vi "4_2_match_per_line.vi"(11 "String":string) -> (1 "Numeric":i32, 3 "match substring":string)   [LabVIEW 2021, in "2023.lvlib"]
uses:
  2023.lvlib
  Program Files (x86)/National Instruments/LabVIEW 2023/user.lib/_OpenG.lib/array/array.llb/Search 1D Array (I32)__ogtk.vi
  Program Files (x86)/National Instruments/LabVIEW 2023/user.lib/_OpenG.lib/array/array.llb/Delete Elements from 1D Array (I32)__ogtk.vi
  Program Files (x86)/National Instruments/LabVIEW 2023/user.lib/_OpenG.lib/array/array.llb/Remove Duplicates from 1D Array (I32)__ogtk.vi
panel:
  out "array w/ subset deleted":i32[](array[numeric])
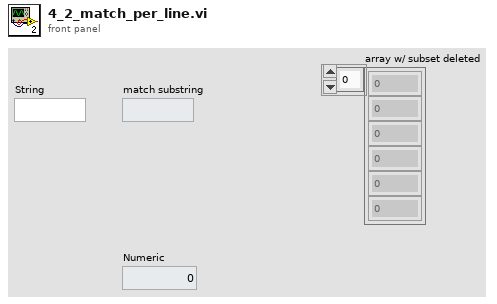
[diagram p1: front panel]
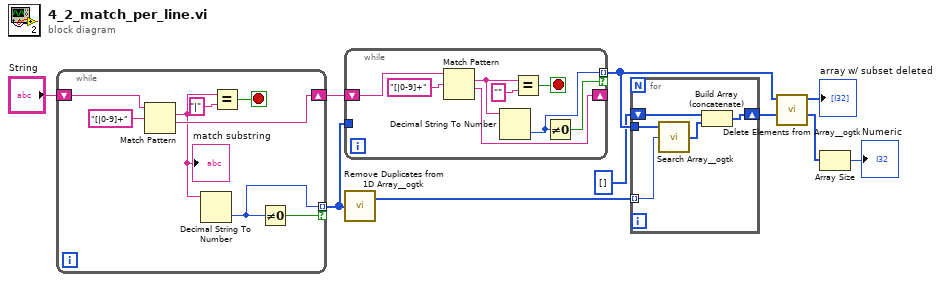
[diagram p0: block diagram]
diagram:
  n1 = while {
    shift-right: [w16] -> w3
    shift-left: "String" -> [w17]
    tunnel: [w12] -> w8 mode=indexing if=w11
    stop <- w13 stop-if-true
    n2 = Match Pattern(string=w17, regular expression="[|0-9]+") -> (match substring=w14:string, after substring=w16:string)  [unwired: 1 in, 2 out]
    "match substring" <- w14
    n3 = Decimal String To Number(string=w14) -> (number=w12:i32)  [unwired: 2 in, 1 out]
    n4 = Equal?(x=w14, y="|") -> (x = y?=w13:bool)
    n5 = Not Equal To 0?(x=w12) -> (x != 0?=w11:bool)
  }
  n6 = while {
    shift-right: [w24] -> _
    shift-left: w3 -> [w25]
    tunnel: [w19] -> w7 mode=indexing if=w20
    tunnel: w8 -> [_]
    stop <- w21 stop-if-true
    n7 = Match Pattern(string=w25, regular expression="[|0-9]+") -> (match substring=w22:string, after substring=w24:string)  [unwired: 1 in, 2 out]
    n8 = Decimal String To Number(string=w22) -> (number=w19:i32)  [unwired: 2 in, 1 out]
    n9 = Equal?(x=w22, y="") -> (x = y?=w21:bool)
    n10 = Not Equal To 0?(x=w19) -> (x != 0?=w20:bool)
  }
  n11 = call-poly "Remove Duplicates from 1D Array__ogtk.vi"("Input Array"=w8) -> ("Output Array"=w6:i32[])  [unwired: 1 out]
  n12 = for {
    tunnel: w6 -> [w31] mode=indexing
    shift-right: [w29] -> w5
    shift-left: i32[] [] -> [w28]
    tunnel: w7 -> [w27]
    n13 = call-poly "Search Array__ogtk.vi"("Array"=w27, "Element Data"=w31) -> ("Indices of Elements"=w30:i32[])  [unwired: 7 in]
    n14 = Build Array (concatenate)(w28, w30) -> (w29:i32[])
  }
  n15 = call-poly "Delete Elements from Array__ogtk.vi"("indices"=w5, "array"=w7) -> ("deleted elements"=w9:i32[], "array w/ subset deleted"=→"array w/ subset deleted":i32[])  [unwired: 8 in]
  n16 = Array Size(array=w9) -> (size(s)=→"Numeric":i32)
